vi "Module_IORead.vi"(6 "IOName-LineName":cluster{"IOName":string, "DAQmxChannel":tag}[](array[cluster])=[{"IOName"="EMG-1", "DAQmxChannel"="PXI2Slot3/port0/line0"}, {"IOName"="READY", "DAQmxChannel"="PXI2Slot3/port0/line1"}], 7 "IORead_Cmd":T3, 8 "error in (no error)":errorcluster caption="エラー入力", 9 "IONames":string[](array[string]), 10 "IOName":string, 11 "IO_State(ForceSet)":T1(array[cluster])) -> (0 "error out":errorcluster caption="エラー出力", 1 "ON/OFF(Plural)":bool[](array[boolean]), 2 "ON/OFF":bool, 3 "IO_State":T1(array[cluster]))   [LabVIEW 2018]
doc: "Module_IORead.vi\nIO信号を初期化、読み取り、クローズ処理する。\n\n◆IORead_Cmd=Init\n　IO信号読み取り用DIを初期化処理する。\n　その際に入力のIO名とライン名の対応付けを保持する。\n　・Input：IOName-LineName\n\n◆IORead_Cmd=Read\n　現在のIO信号(IN)の状態を読み出す。\n　･Output：IO_State\n\n◆IORead_Cmd=Check\n　Readｺﾏﾝﾄﾞで読み取ったIO信号から、指定のIO名の信号の状態を読みだす。\n　(もしくはForceSetｺﾏﾝﾄﾞで設定した信号から、指定のIO名信号を読み出す。)\n　･Input：IOName\n　･Output：ON/OFF\n\n◆IORead_Cmd=Check(Plural)\n　Readｺﾏﾝﾄﾞで読み取ったIO信号から、指定のIO名(複数)の信号の状態を読みだす。\n　(もしくはForceSetｺﾏﾝﾄﾞで設定した信号から、指定のIO名信号を読み出す。)\n　･Input：IONames\n　･Output：ON/OFF(Plural)\n\n◆IORead_Cmd=Close\n　IO信号読み取り用DIをクローズ処理する。\n\n◆IORead_Cmd=ForceSet\n　IO信号の読み取り値を入力の値に強制的に設定する。\n　･Input：IO_State(ForceSet)"
uses:
  Ctl_IOReadCommand.ctl
  <vilib>/DAQmx/read.llb/DAQmx Read (Digital 1D Bool NChan 1Samp 1Line).vi
  <vilib>/DAQmx/create/channels.llb/DAQmx Create Channel (DI-Digital Input).vi
  <vilib>/DAQmx/miscellaneous.llb/DAQmx Fill In Error Info.vi
panel:
  in  "IOState":T2
  # "Local"
  # "Input"
  # "Output"
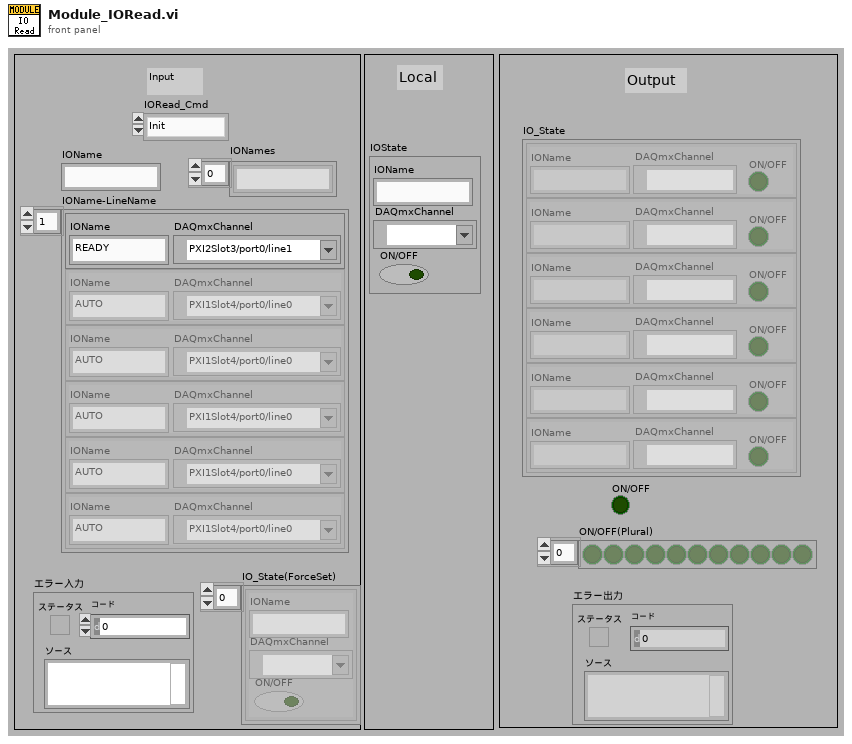
[diagram p1: front panel]
types:
  T1 = cluster{"IOName":string, "DAQmxChannel":tag, "ON/OFF":bool}[]
  T2 = cluster{"IOName":string, "DAQmxChannel":tag, "ON/OFF":bool}
  T3 = typedef "Ctl_IOReadCommand.ctl" = enum16{"Init", "Read", "Check", "Check(Plural)", "Close", "ForceSet"}
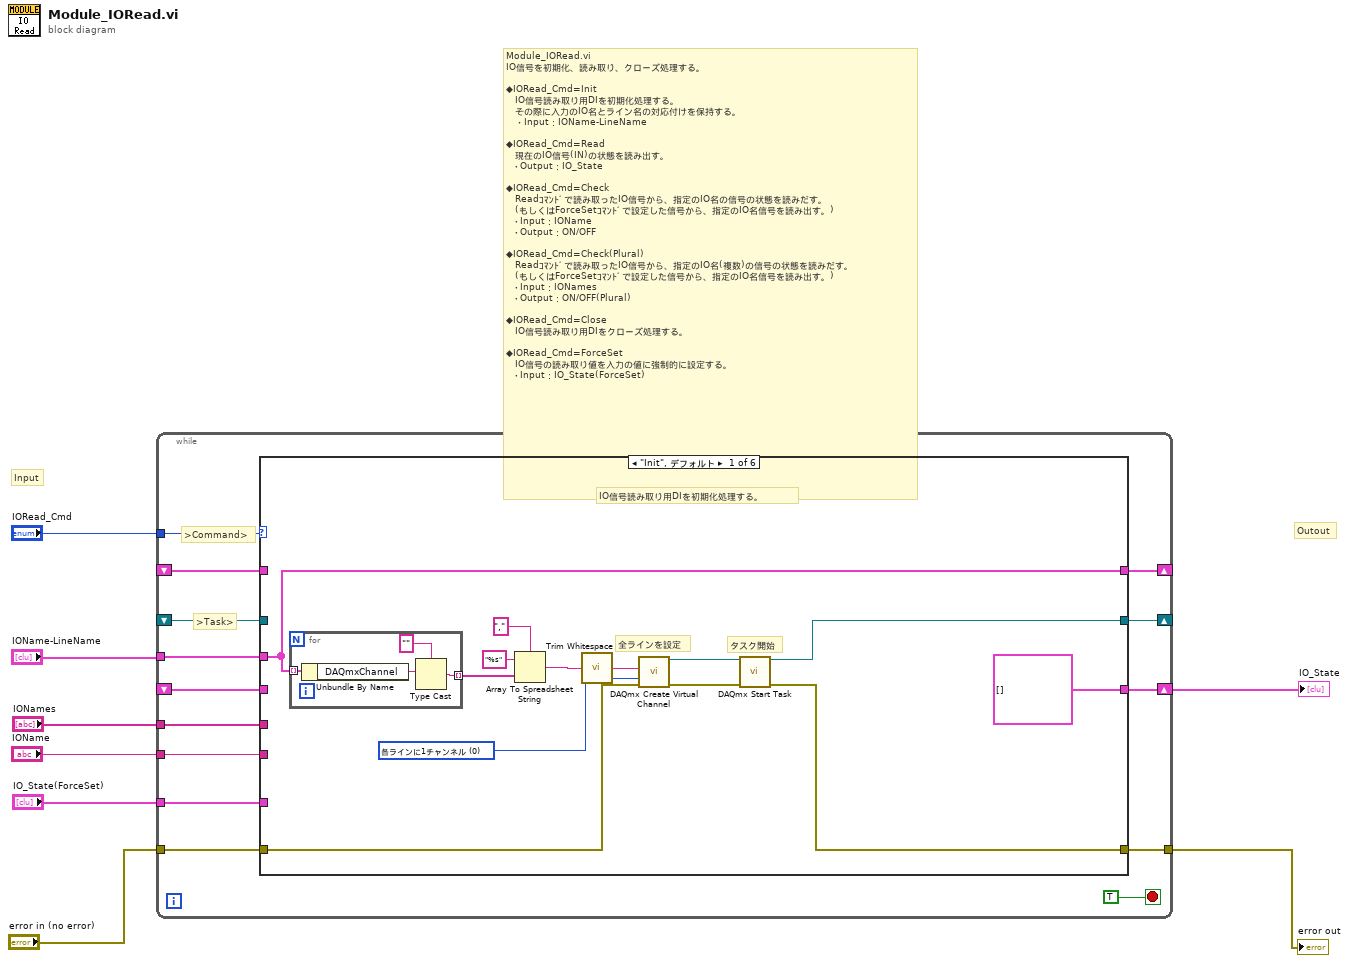
[diagram p0: block diagram]
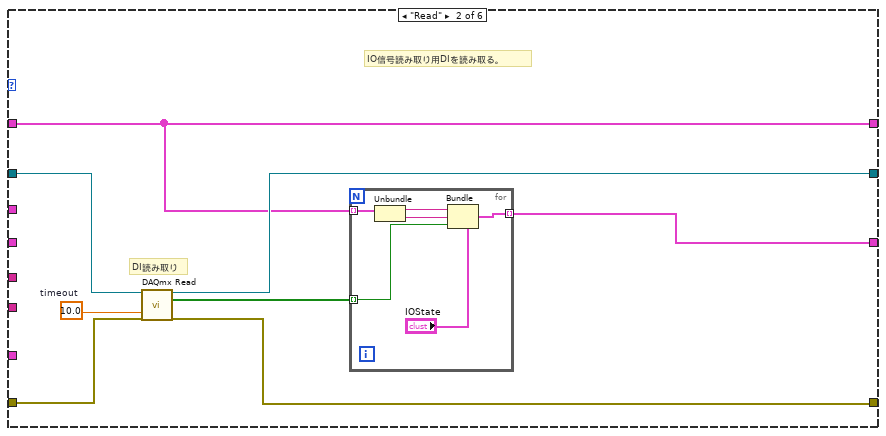
[diagram p2: hidden frame]
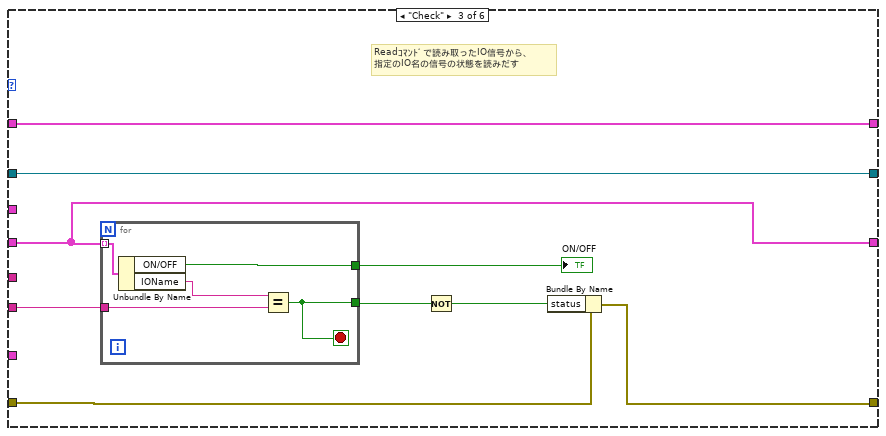
[diagram p3: hidden frame]
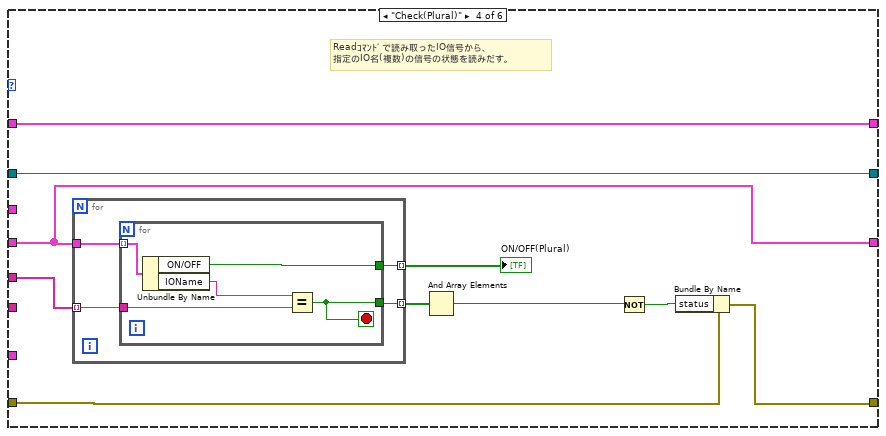
[diagram p4: hidden frame]
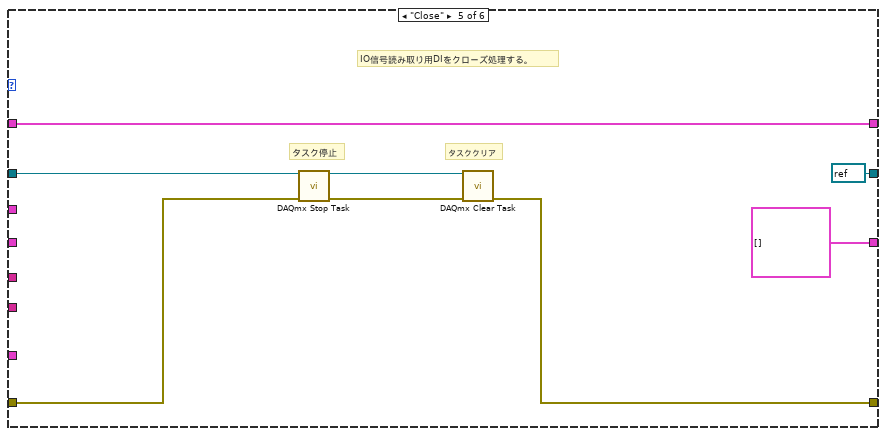
[diagram p5: hidden frame]
diagram:
  # "Module_IORead.vi\nIO信号を初期化、読み取り、クローズ処理する。\n\n◆IORead_Cmd=Init\n　IO信号読み取り用DIを初期化処理する。\n　その際に入力のIO名とライン名の対応付けを保持する。\n　・Input：IOName-LineName\n\n◆IORead_Cmd=Read\n　現在のIO信号(IN)の状態を読み出す。\n　･Output：IO_State\n\n◆IORead_Cmd=Check\n　Readｺﾏﾝﾄﾞで読み取ったIO信号から、指定のIO名の信号の状態を読みだす。\n　(もしくはForceSetｺﾏﾝﾄﾞで設定した信号から、指定のIO名信号を読み出す。)\n　･Input：IOName\n　･Output：ON/OFF\n\n◆IORead_Cmd=Check(Plural)\n　Readｺﾏﾝﾄﾞで読み取ったIO信号から、指定のIO名(複数)の信号の状態を読みだす。\n　(もしくはForceSetｺﾏﾝﾄﾞで設定した信号から、指定のIO名信号を読み出す。)\n　･Input：IONames\n　･Output：ON/OFF(Plural)\n\n◆IORead_Cmd=Close\n　IO信号読み取り用DIをクローズ処理する。\n\n◆IORead_Cmd=ForceSet\n　IO信号の読み取り値を入力の値に強制的に設定する。\n　･Input：IO_State(ForceSet)"
  # "Outout"
  # "Input"
  n1 = while {
    tunnel: "error in (no error)" -> [w22]
    tunnel: [w21] -> w1
    tunnel: "IORead_Cmd" -> [w20]
    shift-right: [w18] -> _
    shift-left: _ -> [w17]
    tunnel: "IOName-LineName" -> [w16]
    shift-right: [w11] -> w5
    shift-left: _ -> [w15]
    tunnel: "IOName" -> [w14]
    shift-right: [w13] -> _
    shift-left: _ -> [w12]
    tunnel: "IO_State(ForceSet)" -> [w10]
    tunnel: "IONames" -> [w9]
    stop <- TRUE stop-if-true
    # ">Task>"
    # ">Command>"
    n2 = case shown="\"Init\", デフォルト" w20 {
      tunnel: w22 -> [w35 w46 w58 w75 w94 w95]
      tunnel: [w26 w42 w57 w74 w88 w95] -> w21
      tunnel: [w31 w45 w62 w77 refnum<k21> refnum ("task out") w97] -> w18
      tunnel: w17 -> [_ w47 w62 w77 w93 w97]
      tunnel: w16 -> [w27 _ _ _ _ _]
      tunnel: [T1 [] w41 w55 w72 T1 [] w96] -> w11
      tunnel: w15 -> [_ _ w55 w72 _ _]
      tunnel: w14 -> [_ _ w60 _ _ _]
      tunnel: [w27 w40 w61 w76 w89 w98] -> w13
      tunnel: w12 -> [_ w40 w61 w76 w89 w98]
      tunnel: w10 -> [_ _ _ _ _ w96]
      tunnel: w9 -> [_ _ _ w71 _ _]
      frame "Init", Default {
        w34 = 0 items=["各ラインに1チャンネル", "全てのラインに1チャンネル"] ("line grouping")
        # "全ラインを設定"
        # "IO信号読み取り用DIを初期化処理する。"
        # "タスク開始"
        n3 = for {
          tunnel: w27 -> [w39] mode=indexing
          tunnel: [w36] -> w28 mode=indexing
          n4 = Unbundle By Name(w39) -> ("DAQmxChannel"=w38:tag)
          n5 = Type Cast(type="" ("タイプ"), x=w38) -> (*(type *) &x=w36:string)
        }
        n6 = Array To Spreadsheet String(delimiter (Tab)="," ("デリミタ（タブ）"), array=w28, 3:"%s" ("形式文字列")) -> (spreadsheet string=w24:string)
        n7 = call <vilib>:"Trim Whitespace.vi"("string"=w24) -> ("trimmed string"=w23:string)  [unwired: 1 in]
        n8 = call-poly <vilib>:"DAQmx Create Virtual Channel.vi"("lines"=w23, "line grouping"=w34, "error in"=w35) -> ("task out"=w32:refnum<k21>, "error out"=w33:errorcluster)  [unwired: 11 in]
        n9 = call <vilib>:"DAQmx Start Task.vi"("task/channels in"=w32, "error in"=w33) -> ("task out"=w31:refnum<k21>, "error out"=w26:errorcluster)  [unwired: 12 in]
      }
      frame "Read" {
        w44 = 10.0  # timeout
        # "IO信号読み取り用DIを読み取る。"
        # "DI読み取り"
        n10 = call-poly <vilib>:"DAQmx Read.vi"("task/channels in"=w47, "timeout"=w44, "error in"=w46) -> ("task out"=w45:refnum<k21>, "data"=w43:bool[], "error out"=w42:errorcluster)  [unwired: 10 in]
        n11 = for {
          tunnel: w40 -> [w50] mode=indexing
          tunnel: w43 -> [w53] mode=indexing
          tunnel: [w52] -> w41 mode=indexing
          n12 = Unbundle(w50) -> ("IOName"=w49:string, "DAQmxChannel"=w48:tag)
          n13 = Bundle(cluster="IOState", "IOName"=w49, "DAQmxChannel"=w48, "ON/OFF"=w53) -> (w52:T2)
        }
      }
      frame "Check" {
        # "Readｺﾏﾝﾄﾞで読み取ったIO信号から、\n指定のIO名の信号の状態を読みだす"
        n14 = for {
          tunnel: w55 -> [w67] mode=indexing
          tunnel: w60 -> [w66]
          tunnel: [w63] -> w59
          tunnel: [w65] -> w54
          stop <- w63 stop-if-true
          n15 = Unbundle By Name(w67) -> ("ON/OFF"=w65:bool, "IOName"=w64:string)
          n16 = Equal?(x=w64, y=w66) -> (x = y?=w63:bool)
        }
        "ON/OFF" <- w54
        n17 = Not(x=w59) -> (.not. x?=w56:bool)
        n18 = Bundle By Name(cluster=w58, "status"=w56) -> (w57:errorcluster)
      }
      frame "Check(Plural)" {
        # "Readｺﾏﾝﾄﾞで読み取ったIO信号から、\n指定のIO名(複数)の信号の状態を読みだす。"
        n19 = for {
          tunnel: [w81] -> w70 mode=indexing
          tunnel: w72 -> [w80]
          tunnel: w71 -> [w79] mode=indexing
          tunnel: [w78] -> w68 mode=indexing
          n20 = for {
            tunnel: w80 -> [w86] mode=indexing
            tunnel: [w84] -> w81
            tunnel: [w85] -> w78
            tunnel: w79 -> [w83]
            stop <- w84 stop-if-true
            n21 = Unbundle By Name(w86) -> ("ON/OFF"=w85:bool, "IOName"=w82:string)
            n22 = Equal?(x=w82, y=w83) -> (x = y?=w84:bool)
          }
        }
        "ON/OFF(Plural)" <- w68
        n23 = And Array Elements(Boolean array=w70) -> (logical AND=w69:bool)
        n24 = Not(x=w69) -> (.not. x?=w73:bool)
        n25 = Bundle By Name(cluster=w75, "status"=w73) -> (w74:errorcluster)
      }
      frame "Close" {
        # "IO信号読み取り用DIをクローズ処理する。"
        # "タスククリア"
        # "タスク停止"
        n26 = call <vilib>:"DAQmx Stop Task.vi"("task/channels in"=w93, "error in"=w94) -> ("task out"=w92:refnum<k21>, "error out"=w91:errorcluster)  [unwired: 12 in]
        n27 = call <vilib>:"DAQmx Clear Task.vi"("task in"=w92, "error in"=w91) -> ("error out"=w88:errorcluster)  [unwired: 13 in]
      }
      frame "ForceSet" {
        # "IO信号の読み取り値を入力の値に強制的に設定する。"
      }
    }
  }
  "error out" <- w1
  "IO_State" <- w5
